vi "CL3IF_GetLightWaveform.vi"(8 "error in":errorcluster {"code" format="%x"}, 9 "peakNo":T1 items=["CL3IF_PEAKNO_01"=1, "CL3IF_PEAKNO_02"=2, "CL3IF_PEAKNO_03"=4, "CL3IF_PEAKNO_04"=8], 10 "headNo":u8, 11 "deviceId":i32) -> (0 "error out":errorcluster {"code" format="%x"}, 2 "waveData":u16[](array[numeric]))   [LabVIEW 2020, in "Keyence CL-3000.lvlib"]
doc: "This function gets the received light waveform data."
uses:
  Keyence CL-3000.lvlib
  enums/CL3IF_PEAKNO.ctl
  Private/enums/Function Name.ctl
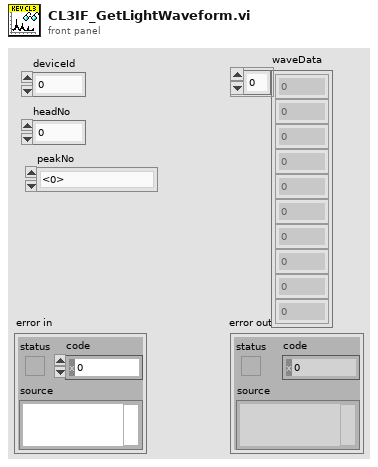
[diagram p1: front panel]
types:
  T1 = typedef "Keyence CL-3000.lvlib/CL3IF_PEAKNO.ctl" = u16
  T2 = typedef "Keyence CL-3000.lvlib/Function Name.ctl" = enum16{"Initialize", "Close", "CL3IF_GetMeasurementData", "CL3IF_GetTrendIndex", "CL3IF_GetTrendData", "CL3IF_GetStorageIndex", "CL3IF_GetStorageData", "CL3IF_AutoZeroMulti", "CL3IF_AutoZeroGroup", "CL3IF_TimingMulti", "CL3IF_TimingGroup", "CL3IF_ResetMulti", "CL3IF_ResetGroup", "CL3IF_LightControl", "CL3IF_MeasurementControl", "CL3IF_SwitchProgram", "CL3IF_GetProgramNo", "CL3IF_StartStorage", "CL3IF_StopStorage", "CL3IF_ClearStorageData", "CL3IF_GetPulseCount", "CL3IF_ResetPulseCount", "CL3IF_GetLightWaveform"}
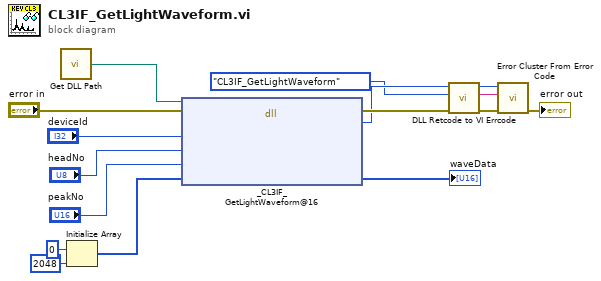
[diagram p0: block diagram]
diagram:
  n1 = call "Get DLL Path.vi"() -> ("DLL Path"=w12:path)  [unwired: 1 in]
  n2 = Initialize Array(u16 0, 2048) -> (w4:u16[])
  n3 = dll-call lib="C:/Program Files (x86)/National Instruments/LabVIEW 2018/instr.lib/Keyence CL-3000/CL3_IF.dll" fn="_CL3IF_GetLightWaveform@16"(path in=w12, error in="error in", "deviceId"="deviceId", "HeadNo"="headNo", "PeakNo"="peakNo", "WaveData"=w4) -> (error out=w11:errorcluster, "RC"=w3:i32, "WaveData"=→"waveData":u16[])  [unwired: 4 in, 1 out]
  n4 = call "DLL Retcode to VI Errcode.vi"("error in (no error)"=w11, "Function Name"=Function_Name."CL3IF_GetLightWaveform", "DLL Retcode"=w3) -> ("error out"=w16:errorcluster, "ErrorMessage"=w2:string, "VI Errcode"=w15:i32)  [unwired: 6 in]
  n5 = call <vilib>:"Error Cluster From Error Code.vi"("error in (no error)"=w16, "error message (\"\")"=w2, "error code (0)"=w15) -> ("error out"=→"error out":errorcluster)  [unwired: 6 in]
